vi "StateReverse_Init.vi"(0 "object in":refnum<class "StateReverse.lvclass">, 1 "StatesData":T4[](array[typedef]), 5 "error in (no error)":errorcluster, 6 "StateStrings":string[](array[string]), 8 "ExitStates":string[](array[string])) -> (14 "object out":refnum<class "StateReverse.lvclass">, 19 "error out":errorcluster)   [LabVIEW 2020, in "StateReverse.lvclass"]
uses:
  <resource>/Framework/Providers/Open_GDS/UML/StateReverse_class/StateReverse.lvclass
  <resource>/Framework/Providers/Open_GDS/ClassProviders/Common/ScriptingFunctions/Scripting_PastThroughObjectType.ctl
  <resource>/Framework/Providers/Open_GDS/ClassProviders/Common/ScriptingFunctions/Scripting_ObjectType.ctl
  <resource>/Framework/Providers/Open_GDS/UML/StateReverse_class/StateDetails.ctl
  <resource>/Framework/Providers/Open_GDS/UML/StateReverse_class/NextStateAction.ctl
  <resource>/Framework/Providers/Open_GDS/UML/StateReverse_class/StateAction.ctl
  <resource>/Framework/Providers/Open_GDS/UML/StateReverse_class/StateReverse.lvclass/StateReverse.ctl
  <resource>/Framework/Providers/Open_GDS/ClassProviders/Common/ScriptingFunctions/Scripting.lvclass
panel:
  out "Array":T1[](array[typedef])
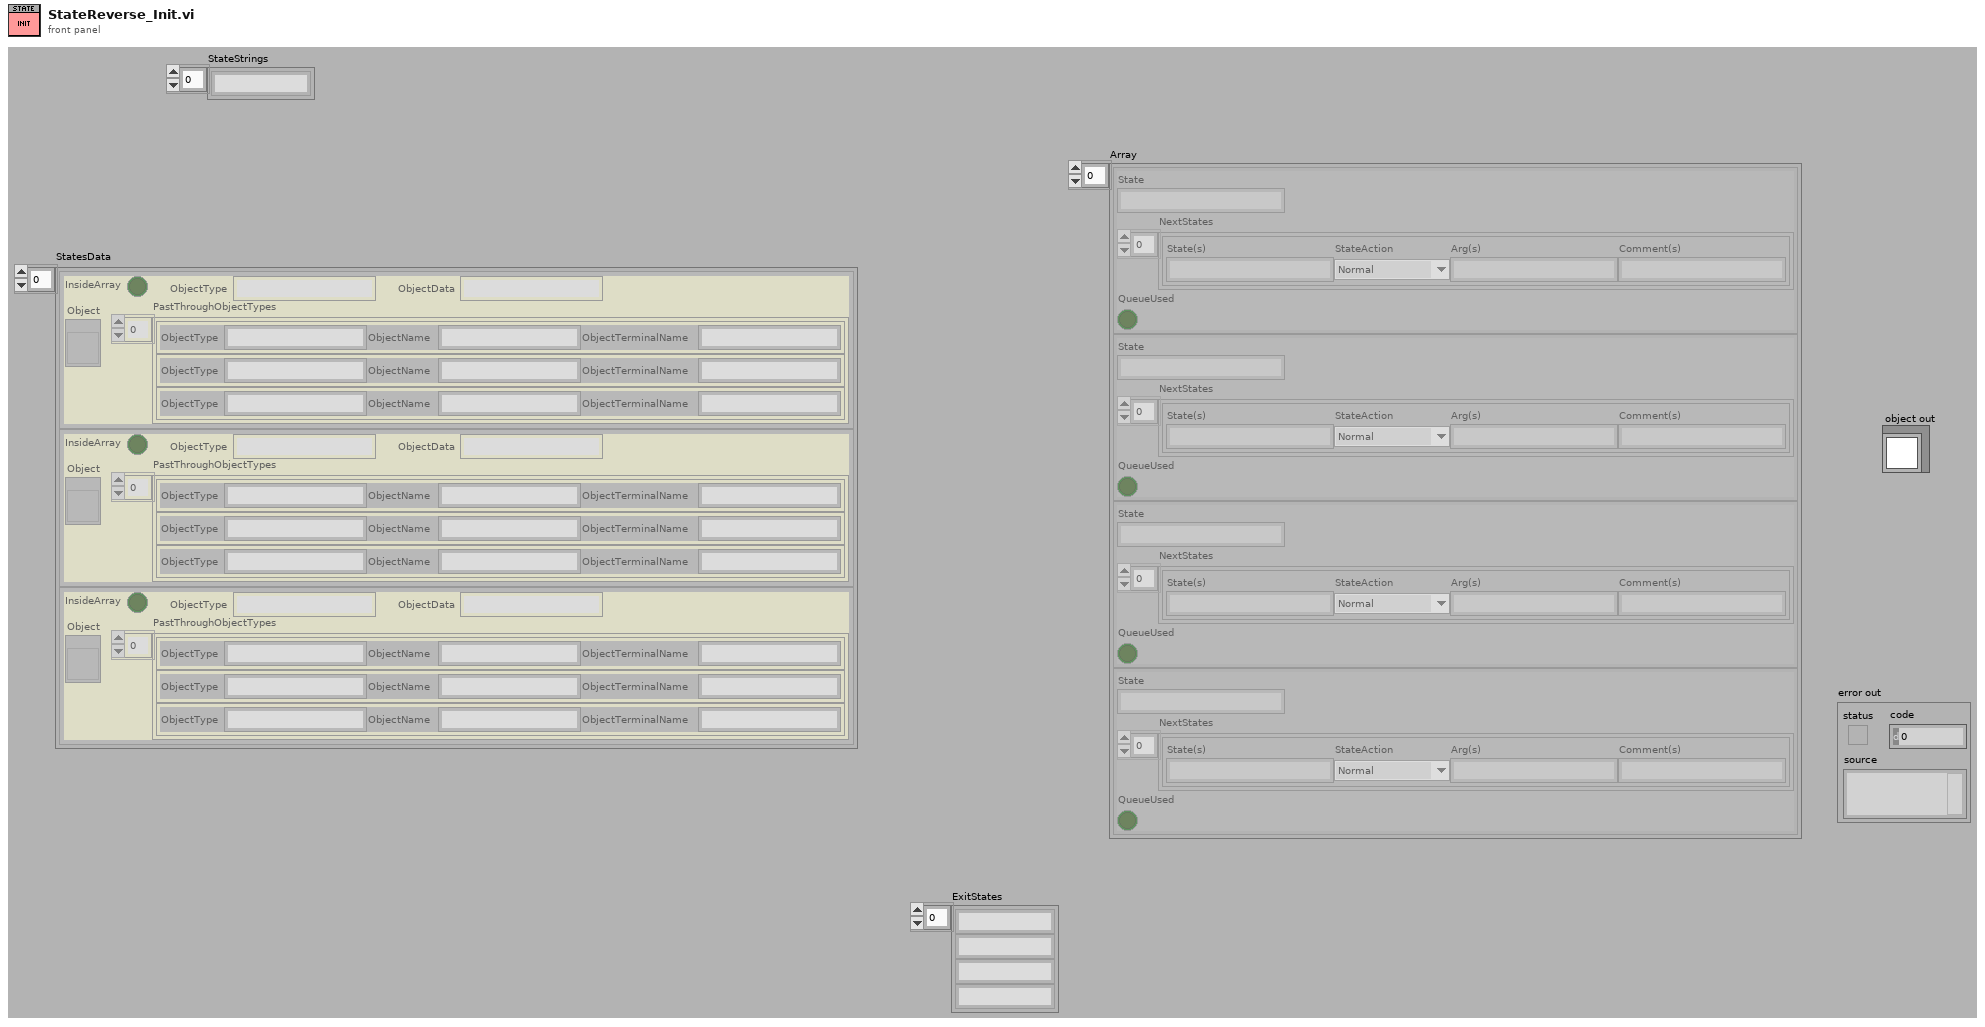
[diagram p1: front panel]
types:
  T1 = typedef "StateReverse.lvclass/StateDetails.ctl" = cluster{"State":string, "NextStates":T2[], "QueueUsed":bool}
  T2 = typedef "StateReverse.lvclass/NextStateAction.ctl" = cluster{"State(s)":string, "StateAction":T3, "Arg(s)":string, "Comment(s)":string}
  T3 = typedef "StateReverse.lvclass/StateAction.ctl" = enum16{"Normal", "AddInBeggining", "AddInEnd", "AddIfNothingInQueue"}
  T4 = typedef "Scripting.lvclass/Scripting_PastThroughObjectType.ctl" = cluster{"Object":refnum<vi>, "InsideArray":bool, "PastThroughObjectTypes":T5[], "ObjectType":string, "ObjectData":string}
  T5 = typedef "Scripting_ObjectType.ctl" = cluster{"ObjectType":string, "ObjectName":string, "ObjectTerminalName":string}
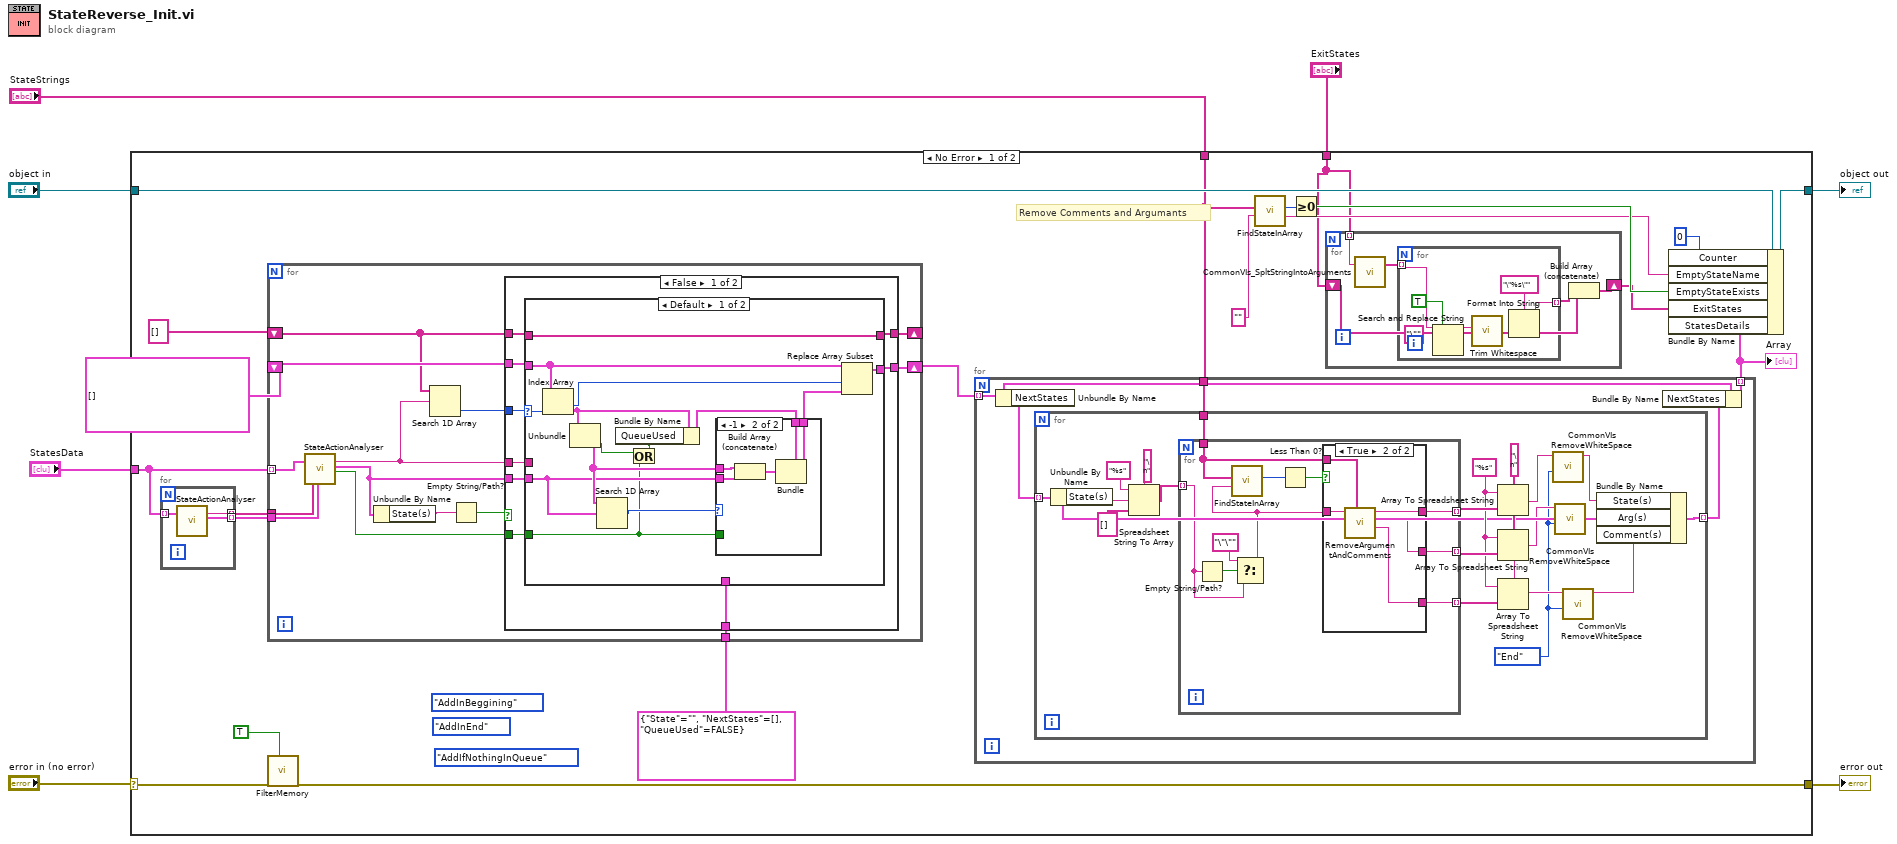
[diagram p0: block diagram]
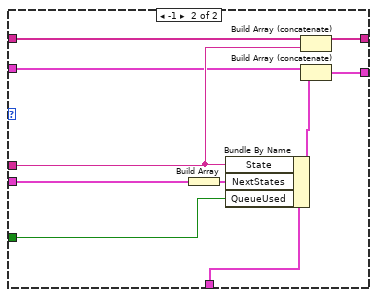
[diagram p4: hidden frame]
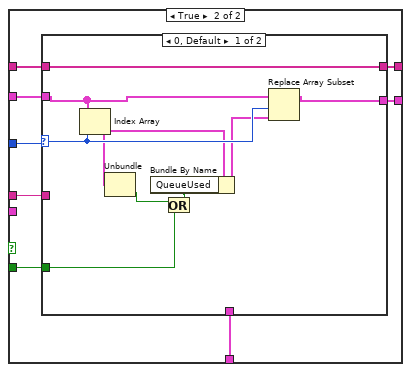
[diagram p5: hidden frame]
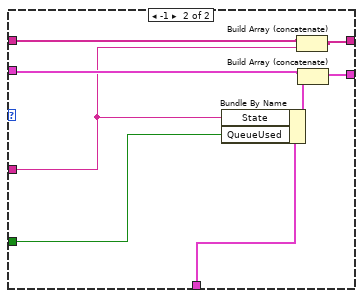
[diagram p6: hidden frame]
diagram:
  n1 = case shown="No Error" "error in (no error)" {
    selector: "error in (no error)" -> [w13 w162]
    tunnel: "object in" -> [w28 w163]
    tunnel: [w27 w163] -> w6
    tunnel: [w12 w162] -> w4
    tunnel: "StatesData" -> [w10 _]
    tunnel: "StateStrings" -> [w19 _]
    tunnel: "ExitStates" -> [w15 _]
    frame No Error {
      (unwired) StateAction."AddIfNothingInQueue" ("StateAction")
      (unwired) StateAction."AddInEnd" ("StateAction")
      (unwired) StateAction."AddInBeggining" ("StateAction")
      # "Remove Comments and Argumants"
      n2 = for {
        tunnel: w10 -> [w31] mode=indexing
        tunnel: [w30] -> w9 mode=indexing
        tunnel: [w29] -> w8 mode=indexing
        n3 = call <resource>:"StateActionAnalyser.vi"("FoundObjectOnWire"=w31) -> ("CaseState"=w30:string, "StateAction"=w29:T2)  [unwired: 16 in, 1 out]
      }
      n4 = for {
        tunnel: w10 -> [w93] mode=indexing
        tunnel: T1 {"State"="", "NextStates"=[], "QueueUsed"=FALSE} ("StateDetails") -> [w98]
        shift-right: [w96] -> _
        shift-left: string[] [] -> [w94]
        shift-right: [w97] -> w23
        shift-left: T1[] [] -> [w95]
        tunnel: w9 -> [w86]
        tunnel: w8 -> [w85]
        n5 = call <resource>:"StateActionAnalyser.vi"("FoundObjectOnWire"=w93, "CaseStatesIn(IgnoredIfNotWired)"=w86, "StateActionIn(IgnoredIfNotWired)"=w85) -> ("CaseState"=w92:string, "StateAction"=w91:T2, "Linked to the Parse State Queue VI"=w87:bool)  [unwired: 14 in]
        n6 = Unbundle By Name(w91) -> ("State(s)"=w89:string)
        n7 = Search 1D Array(1D array=w94, element=w92) -> (index of element=w90:i32)  [unwired: 1 in]
        n8 = Empty String/Path?(string/path=w89) -> (empty?=w88:bool)
        n9 = case shown="False" w88 {
          tunnel: w98 -> [w107 w138]
          tunnel: [w106 w140] -> w97
          tunnel: [w105 w142] -> w96
          tunnel: w95 -> [w104 w141]
          tunnel: w94 -> [w103 w143]
          tunnel: w92 -> [w102 w139]
          tunnel: w91 -> [w101 _]
          tunnel: w90 -> [w100 w144]
          tunnel: w87 -> [w99 w137]
          frame False {
            n10 = case shown="Default" w100 {
              selector: w100 -> [w114 _]
              tunnel: w107 -> [_ w136]
              tunnel: w103 -> [w120 w135]
              tunnel: w102 -> [_ w134]
              tunnel: [w118 w132] -> w106
              tunnel: [w120 w131] -> w105
              tunnel: w104 -> [w119 w130]
              tunnel: w101 -> [w115 w129]
              tunnel: w99 -> [w108 w127]
              frame Default {
                n11 = Index Array(array=w119, index=w114) -> (element=w112:T1)
                n12 = Unbundle(w112) -> ("NextStates"=w116:T2[], "QueueUsed"=w110:bool)  [unwired: 1 out]
                n13 = Search 1D Array(1D array=w116, element=w115) -> (index of element=w113:i32)  [unwired: 1 in]
                n14 = Or(x=w110, y=w108) -> (x .or. y?=w109:bool)
                n15 = Bundle By Name(cluster=w112, "QueueUsed"=w109) -> (w111:T1)
                n16 = case shown="-1" w113 {
                  tunnel: w111 -> [w121 w126]
                  tunnel: [w121 w124] -> w117
                  tunnel: w116 -> [_ w123]
                  tunnel: w115 -> [_ w122]
                  tunnel: w108 -> [_ _]
                  frame Default {
                  }
                  frame -1 {
                    n17 = Build Array (concatenate)(w123, w122) -> (w125:T2[])
                    n18 = Bundle(cluster=w126, "NextStates"=w125) -> (w124:T1)  [unwired: 2 in]
                  }
                }
                n19 = Replace Array Subset(array=w119, new element=w117, index=w114) -> (w118:T1[])
              }
              frame -1 {
                n20 = Build Array(w129) -> (w128:T2[])
                n21 = Bundle By Name(cluster=w136, "State"=w134, "NextStates"=w128, "QueueUsed"=w127) -> (w133:T1)
                n22 = Build Array (concatenate)(w135, w134) -> (w131:string[])
                n23 = Build Array (concatenate)(w130, w133) -> (w132:T1[])
              }
            }
          }
          frame True {
            n24 = case shown="0, Default" w144 {
              selector: w144 -> [w151 _]
              tunnel: [w153 w160] -> w142
              tunnel: w143 -> [w153 w161]
              tunnel: w141 -> [w150 w158]
              tunnel: [w152 w159] -> w140
              tunnel: w139 -> [_ w156]
              tunnel: w138 -> [_ w157]
              tunnel: w137 -> [w147 w154]
              frame 0, Default {
                n25 = Index Array(array=w150, index=w151) -> (element=w146:T1)
                n26 = Unbundle(w146) -> ("QueueUsed"=w149:bool)  [unwired: 2 out]
                n27 = Or(x=w149, y=w147) -> (x .or. y?=w148:bool)
                n28 = Bundle By Name(cluster=w146, "QueueUsed"=w148) -> (w145:T1)
                n29 = Replace Array Subset(array=w150, new element=w145, index=w151) -> (w152:T1[])
              }
              frame -1 {
                n30 = Bundle By Name(cluster=w157, "State"=w156, "QueueUsed"=w154) -> (w155:T1)
                n31 = Build Array (concatenate)(w161, w156) -> (w160:string[])
                n32 = Build Array (concatenate)(w158, w155) -> (w159:T1[])
              }
            }
          }
        }
      }
      n33 = call <resource>:"FilterMemory.vi"("Reset"=TRUE, "error in (no error)"=w13) -> ("error out"=w12:errorcluster)  [unwired: 6 in, 3 out]
      n34 = for {
        tunnel: w23 -> [w46] mode=indexing
        tunnel: w19 -> [w47]
        tunnel: [w44] -> w22 mode=indexing
        n35 = Unbundle By Name(w46) -> ("NextStates"=w48:T2[])
        n36 = for {
          tunnel: w48 -> [w57] mode=indexing
          tunnel: w47 -> [w68]
          tunnel: [w56] -> w45 mode=indexing
          w49 = enum16{"Begining", "End", "Beg+End", "All"}."End" ("Remove from")
          w59 = "%s" ("format string")
          w60 = "\n" ("delimiter (Tab)")
          n37 = Unbundle By Name(w57) -> ("State(s)"=w67:string)
          n38 = Spreadsheet String To Array(delimiter (Tab)="\n", format string="%s", spreadsheet string=w67, array type (2D Dbl)=string[] []) -> (array=w63:string[])
          n39 = for {
            tunnel: w68 -> [w75]
            tunnel: w63 -> [w70] mode=indexing
            tunnel: [w76] -> w62 mode=indexing
            tunnel: [w74] -> w61 mode=indexing
            tunnel: [w73] -> w58 mode=indexing
            n40 = Empty String/Path?(string/path=w70) -> (empty?=w72:bool)
            n41 = Select(t="\"\"" ("format string"), s=w72, f=w70) -> (s? t:f=w71:string)
            n42 = call <resource>:"FindStateInArray.vi"("TransactionState"=w71, "AllCaseStates"=w75) -> ("index of element"=w78:i32)  [unwired: 7 in, 2 out]
            n43 = Less Than 0?(x=w78) -> (x < 0?=w77:bool)
            n44 = case shown="True" w77 {
              tunnel: w71 -> [w79 w84]
              tunnel: [w79 w83] -> w76
              tunnel: w75 -> [_ w82]
              tunnel: [_ w81] -> w74
              tunnel: [_ w80] -> w73
              frame False {
              }
              frame True {
                n45 = call <resource>:"RemoveArgumentAndComments.vi"("AllCaseStates"=w82, "TransactionStateIn"=w84) -> ("Comment"=w80:string, "Argument"=w81:string, "TransactionStateOut"=w83:string)  [unwired: 7 in]
              }
            }
          }
          n46 = Array To Spreadsheet String(delimiter (Tab)=w60, array=w62, 3:w59) -> (spreadsheet string=w55:string)
          n47 = Array To Spreadsheet String(delimiter (Tab)=w60, array=w61, 3:w59) -> (spreadsheet string=w53:string)
          n48 = Array To Spreadsheet String(delimiter (Tab)=w60, array=w58, 3:w59) -> (spreadsheet string=w51:string)
          n49 = call <resource>:"CommonVIs RemoveWhiteSpace.vi"("Remove from"=w49, "String in"=w55) -> ("String out"=w54:string)  [unwired: 4 in, 1 out]
          n50 = call <resource>:"CommonVIs RemoveWhiteSpace.vi"("Remove from"=w49, "String in"=w53) -> ("String out"=w52:string)  [unwired: 4 in, 1 out]
          n51 = call <resource>:"CommonVIs RemoveWhiteSpace.vi"("Remove from"=w49, "String in"=w51) -> ("String out"=w50:string)  [unwired: 4 in, 1 out]
          n52 = Bundle By Name(cluster=w57, "State(s)"=w54, "Arg(s)"=w52, "Comment(s)"=w50) -> (w56:T2)
        }
        n53 = Bundle By Name(cluster=w46, "NextStates"=w45) -> (w44:T1)
      }
      "Array" <- w22
      n54 = call <resource>:"FindStateInArray.vi"("TransactionState"="", "AllCaseStates"=w19) -> ("CaseStateOut"=w17:string, "index of element"=w20:i32)  [unwired: 7 in, 1 out]
      n55 = Greater Or Equal To 0?(x=w20) -> (x >= 0?=w18:bool)
      n56 = for {
        tunnel: w15 -> [w32] mode=indexing
        shift-right: [w34] -> w16
        shift-left: w15 -> [w33]
        n57 = call <resource>:"CommonVIs_SpltStringIntoArguments.vi"("String"=w32) -> ("splittedString"=w36:string[])  [unwired: 17 in, 1 out]
        n58 = for {
          tunnel: [w38] -> w35 mode=indexing
          tunnel: w36 -> [w37] mode=indexing
          n59 = Search and Replace String(replace all?=TRUE ("replace all? (F)"), input string=w37, search string="\"") -> (result string=w41:string)  [unwired: 1 in, 7 out]
          n60 = call <vilib>:"Trim Whitespace.vi"("string"=w41) -> ("trimmed string"=w39:string)  [unwired: 1 in]
          n61 = Format Into String(format string="\"%s\"", w39) -> (resulting string=w38:string)  [unwired: 2 in, 1 out]
        }
        n62 = Build Array (concatenate)(w35, w33) -> (w34:string[])
      }
      n63 = Bundle By Name(cluster=w28, "Counter"=0, "EmptyStateName"=w17, "EmptyStateExists"=w18, "ExitStates"=w16, "StatesDetails"=w22) -> (w27:refnum<class "StateReverse.lvclass">)
    }
    frame Error {
    }
  }
  "object out" <- w6
  "error out" <- w4
